vi "LesterRocheparcial2.vi"() -> ()   [LabVIEW 2011]
uses:
  LesterRocheparcial2.ctl
panel:
  out "promedio de las temperatura":dbl
  out "temperatura minima":dbl
  out "Temperatura maxima":dbl
  out "Array 2":bool[](array[boolean])
  out "Array":i32[](array[slide]) scale=0.0..60.0
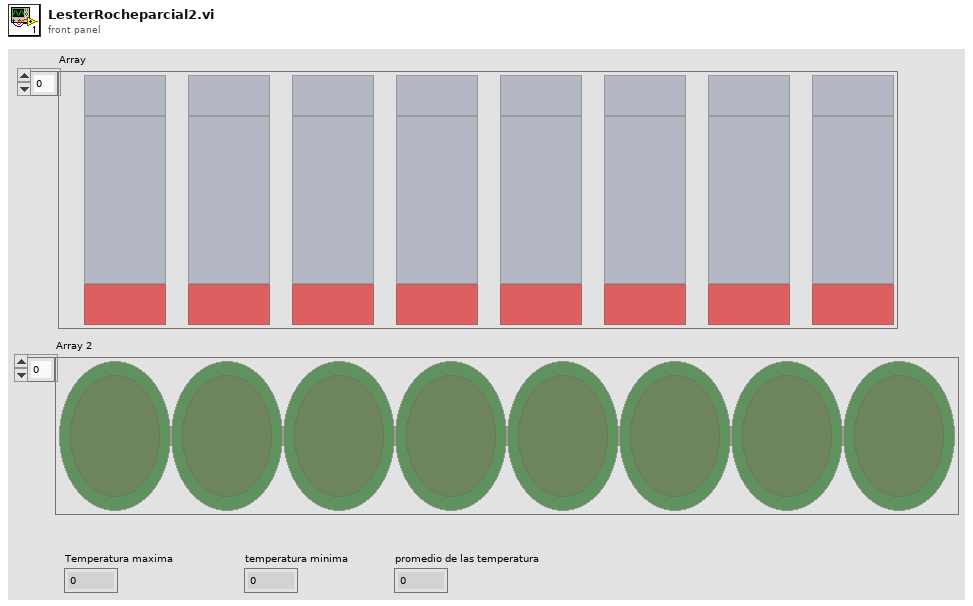
[diagram p1: front panel]
types:
  T1 = typedef "LesterRocheparcial2.ctl" = enum16{"Iniciar arreglos", "rellenar arreglos", "promedio", "maximo y minimo", "encender los led", "finalizar"}
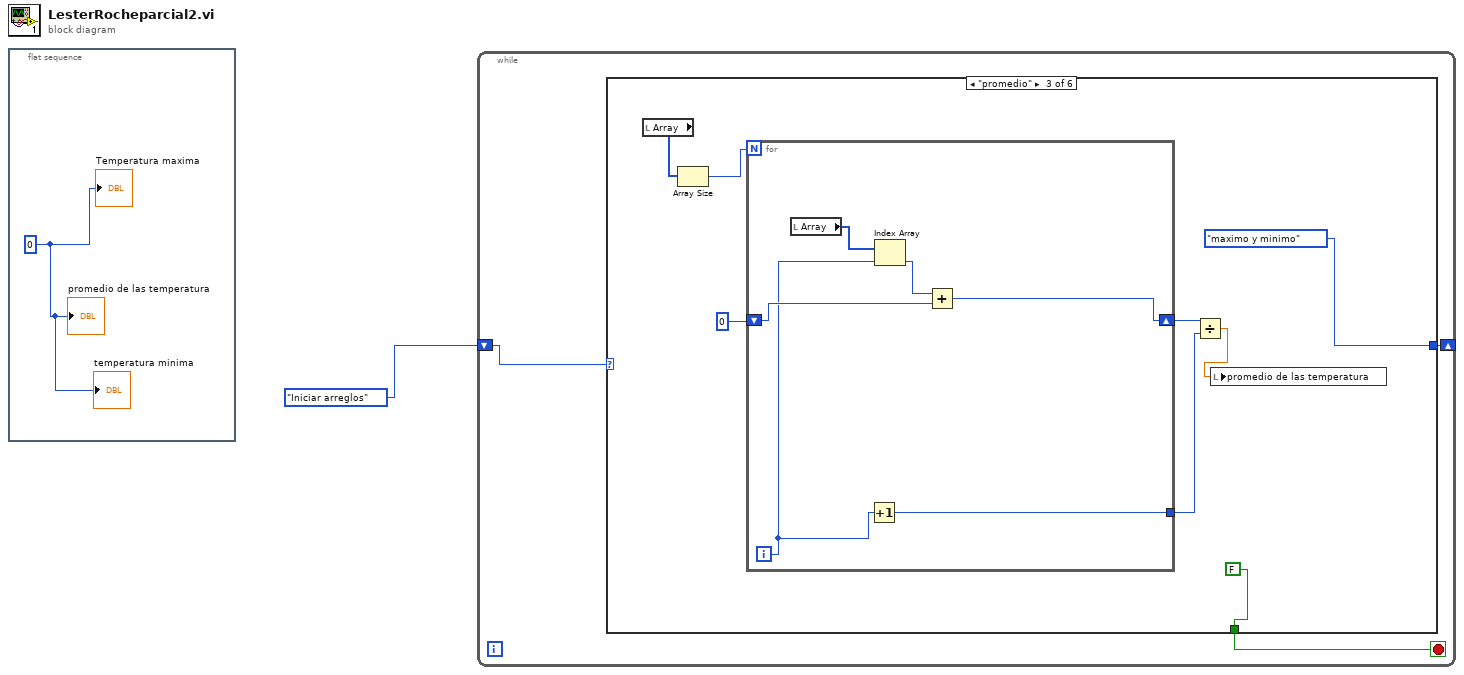
[diagram p0: block diagram]
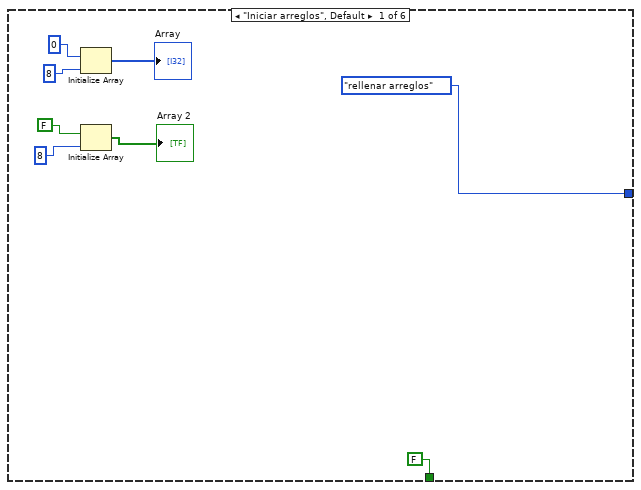
[diagram p2: hidden frame]
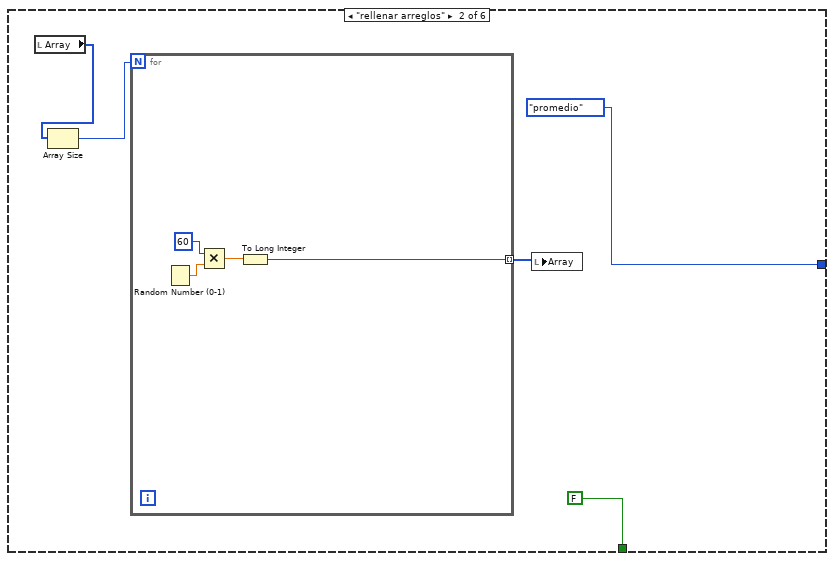
[diagram p3: hidden frame]
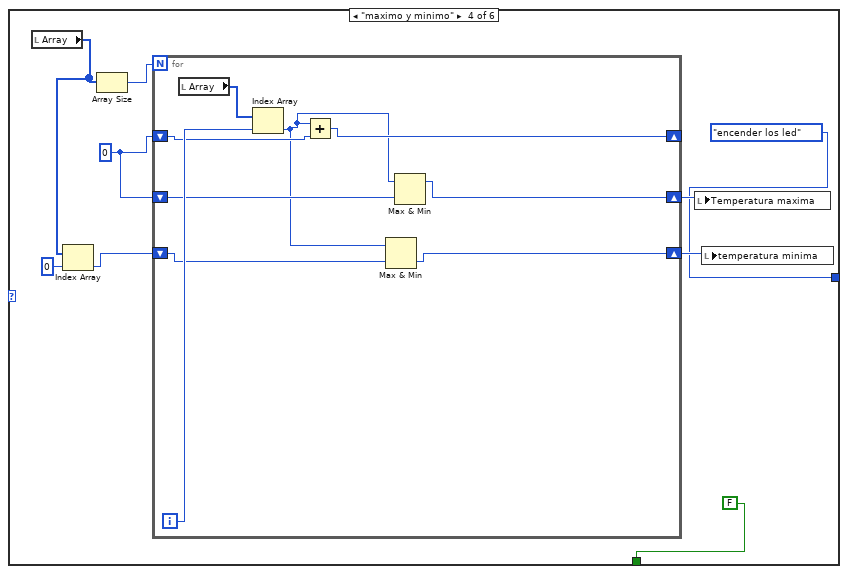
[diagram p4: hidden frame]
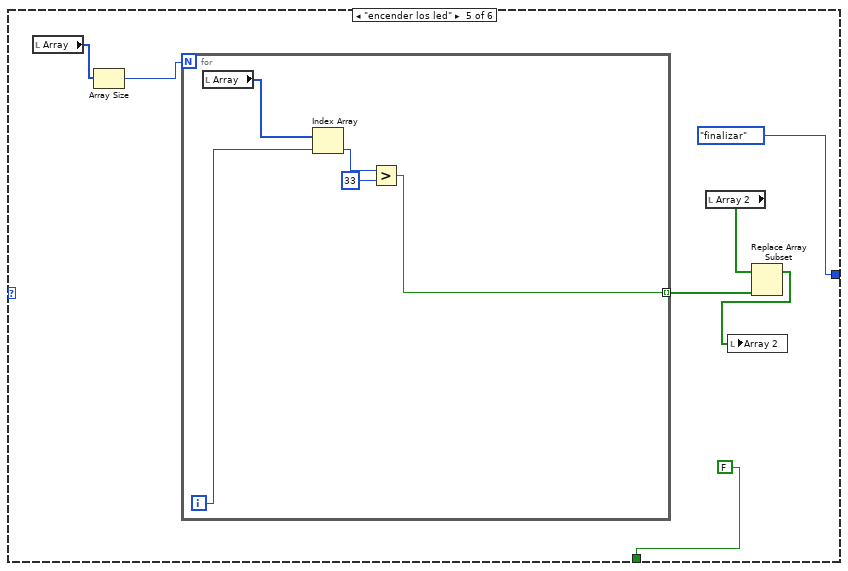
[diagram p5: hidden frame]
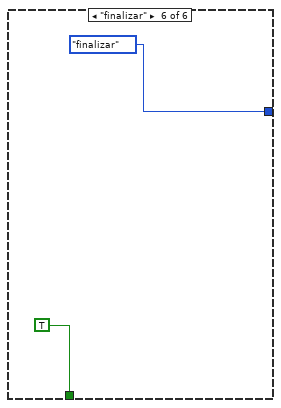
[diagram p6: hidden frame]
diagram:
  n1 = flat-sequence {
    frame #0 {
      w2 = 0
      "temperatura minima" <- w2
      "promedio de las temperatura" <- w2
      "Temperatura maxima" <- w2
    }
  }
  n2 = while {
    shift-right: [w3] -> _
    shift-left: LesterRocheparcial2."Iniciar arreglos" -> [w4]
    stop <- w5 stop-if-true
    n3 = case shown="\"promedio\"" w4 {
      tunnel: [FALSE FALSE FALSE FALSE FALSE TRUE] -> w5
      tunnel: [LesterRocheparcial2."rellenar arreglos" LesterRocheparcial2."promedio" LesterRocheparcial2."maximo y minimo" LesterRocheparcial2."encender los led" LesterRocheparcial2."finalizar" LesterRocheparcial2."finalizar"] -> w3
      frame "Iniciar arreglos", Default {
        n4 = Initialize Array "Initialize Array"(0, 8) -> (→"Array":i32[])
        n5 = Initialize Array(FALSE, 8) -> (→"Array 2":bool[])
      }
      frame "rellenar arreglos" {
        n6 = local read "Array"() -> (w16:i32[])
        n7 = Array Size(array=w16) -> (size(s)=w15:i32)
        n8 = for {
          N: w15 -> [_]
          tunnel: [w19] -> w14 mode=indexing
          n9 = Random Number (0-1)() -> (number: 0 to 1=w21:dbl)
          n10 = Multiply(x=60, y=w21) -> (x*y=w20:dbl)
          n11 = To Long Integer(number=w20) -> (32bit integer=w19:i32)
        }
        n12 = local write "Array"(w14) -> ()
      }
      frame "promedio" {
        n13 = local read "Array"() -> (w30:i32[])
        n14 = Array Size(array=w30) -> (size(s)=w29:i32)
        n15 = for {
          N: w29 -> [_]
          shift-right: [w33] -> w27
          shift-left: 0 -> [w34]
          tunnel: [w32] -> w26
          i -> [w31]
          n16 = local read "Array"() -> (w36:i32[])
          n17 = Increment(x=w31) -> (x+1=w32:i32)
          n18 = Index Array(array=w36, index=w31) -> (element=w35:i32)
          n19 = Add(x=w35, y=w34) -> (x+y=w33:i32)
        }
        n20 = Divide(x=w27, y=w26) -> (x/y=w25:dbl)
        n21 = local write "promedio de las temperatura"(w25) -> ()
      }
      frame "maximo y minimo" {
        w44 = 0
        n22 = local read "Array"() -> (w42:i32[])
        n23 = Index Array(array=w42, index=0) -> (element=w40:i32)
        n24 = Array Size(array=w42) -> (size(s)=w45:i32)
        n25 = for {
          N: w45 -> [_]
          shift-right: [w50] -> w43
          shift-left: w44 -> [w51]
          shift-right: [w47] -> w39
          shift-left: w40 -> [w49]
          shift-right: [w48] -> _
          shift-left: w44 -> [w52]
          i -> [w53]
          n26 = local read "Array"() -> (w54:i32[])
          n27 = Index Array(array=w54, index=w53) -> (element=w46:i32)
          n28 = Add(x=w46, y=w52) -> (x+y=w48:i32)
          n29 = Max & Min(x=w46, y=w49) -> (min(x,y)=w47:i32)  [unwired: 1 out]
          n30 = Max & Min(x=w46, y=w51) -> (max(x,y)=w50:i32)  [unwired: 1 out]
        }
        n31 = local write "Temperatura maxima"(w43) -> ()
        n32 = local write "temperatura minima"(w39) -> ()
      }
      frame "encender los led" {
        n33 = local read "Array"() -> (w61:i32[])
        n34 = Array Size(array=w61) -> (size(s)=w60:i32)
        n35 = for {
          N: w60 -> [_]
          tunnel: [w62] -> w58 mode=indexing
          i -> [w65]
          n36 = local read "Array"() -> (w66:i32[])
          n37 = Index Array(array=w66, index=w65) -> (element=w64:i32)
          n38 = Greater?(x=w64, y=33) -> (0:w62:bool)
        }
        n39 = local read "Array 2"() -> (w59:bool[])
        n40 = Replace Array Subset(array=w59, new element=w58) -> (w57:bool[])  [unwired: 1 in]
        n41 = local write "Array 2"(w57) -> ()
      }
      frame "finalizar" {
      }
    }
  }
